vi "Read Blue1.vi"(8 "error in (no error)":errorcluster, 11 "Laser Enable CMD in":refnum<class "Laser Enable CMD.lvclass">) -> (0 "error out":errorcluster, 2 "Blue1":bool, 3 "Laser Enable CMD out":refnum<class "Laser Enable CMD.lvclass">)   [LabVIEW 2014, in "eCRDS Library.lvlib" / "Laser Enable CMD.lvclass"]
uses:
  Laser Enable CMD.lvclass
  Laser Enable CMD.lvclass/Laser Enable CMD.ctl
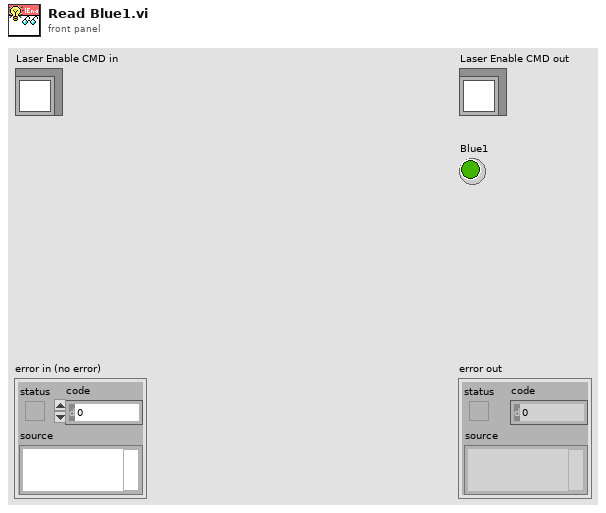
[diagram p1: front panel]
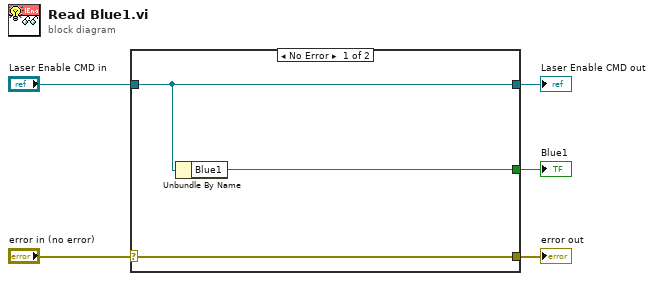
[diagram p0: block diagram]
diagram:
  n1 = case shown="No Error" "error in (no error)" {
    selector: "error in (no error)" -> [w8 w9]
    tunnel: [w8 w9] -> w4
    tunnel: [w7 w10] -> w2
    tunnel: "Laser Enable CMD in" -> [w7 w10]
    tunnel: [w6 _] -> w1
    frame No Error {
      n2 = Unbundle By Name(w7) -> ("Blue1"=w6:bool)
    }
    frame Error {
    }
  }
  "error out" <- w4
  "Laser Enable CMD out" <- w2
  "Blue1" <- w1
